vi "pallindrome elaks.vi"() -> ()   [LabVIEW 2019]
panel:
  out "yes or no":bool
  in  "Numeric":dbl
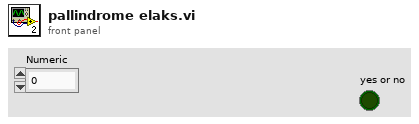
[diagram p1: front panel]
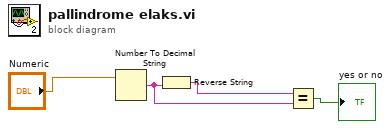
[diagram p0: block diagram]
diagram:
  n1 = Number To Decimal String(number="Numeric") -> (decimal integer string=w2:string)  [unwired: 1 in]
  n2 = Reverse String(1:w2) -> (0:w3:string)
  n3 = Equal?(x=w3, y=w2) -> (x = y?=→"yes or no":bool)
